vi "Write imageRefs.MainImage.vi"(8 "error in (no error)":errorcluster, 10 "Image":T1, 11 "GenericCamera in":refnum<class "GenericCamera.lvclass">) -> (0 "error out":errorcluster, 3 "GenericCamera out":refnum<class "GenericCamera.lvclass">)   [LabVIEW 2013, in "GenericCamera.lvclass"]
uses:
  GenericCamera.lvclass
  <vilib>/vision/Image Controls.llb/IMAQ Image.ctl
  GenericCamera.lvclass/GenericCamera.ctl
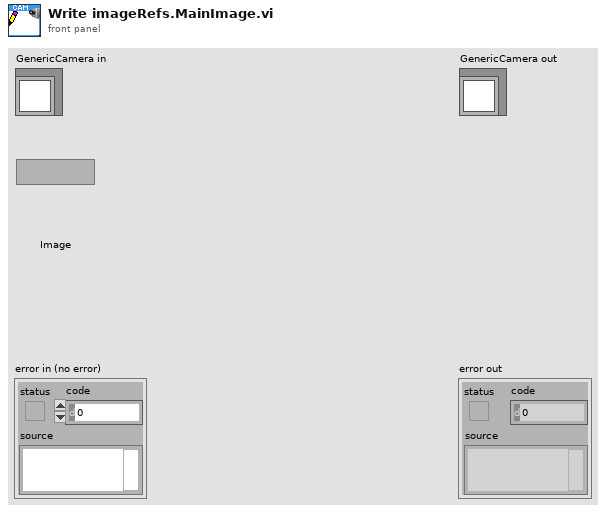
[diagram p1: front panel]
types:
  T1 = typedef "IMAQ Image.ctl" = refnum<image>
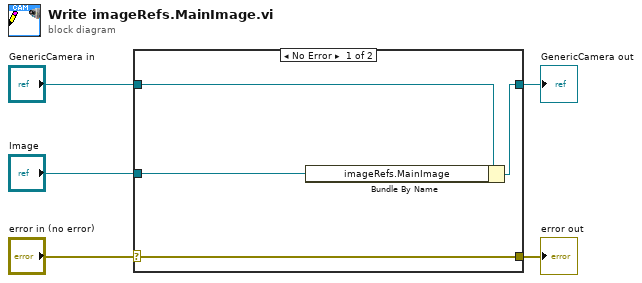
[diagram p0: block diagram]
diagram:
  n1 = case shown="No Error" "error in (no error)" {
    selector: "error in (no error)" -> [w9 w10]
    tunnel: [w9 w10] -> w4
    tunnel: [w7 w11] -> w2
    tunnel: "GenericCamera in" -> [w8 w11]
    tunnel: "Image" -> [w6 _]
    frame No Error {
      n2 = Bundle By Name(cluster=w8, "imageRefs.MainImage"=w6) -> (w7:refnum<class "GenericCamera.lvclass">)
    }
    frame Error {
    }
  }
  "error out" <- w4
  "GenericCamera out" <- w2
